vi "ni579x Write EEPROM.vi"(0 "Register Bus":refnum<class "ni579x Register Bus v1 Host.lvclass">=refnum, 1 "scope":string(combo)="characterization data eeprom", 5 "start address":u32 format="%x", 7 "data":u8[](array[numeric]) format="%x", 11 "Error In":errorcluster) -> (4 "Register Bus (out)":refnum<class "ni579x Register Bus v1 Host.lvclass">, 15 "Error Out":errorcluster)   [LabVIEW 2013]
uses:
  <instrlib>/ni579x/Register Bus/v1/Host/ni579x Register Bus v1 Host.lvclass
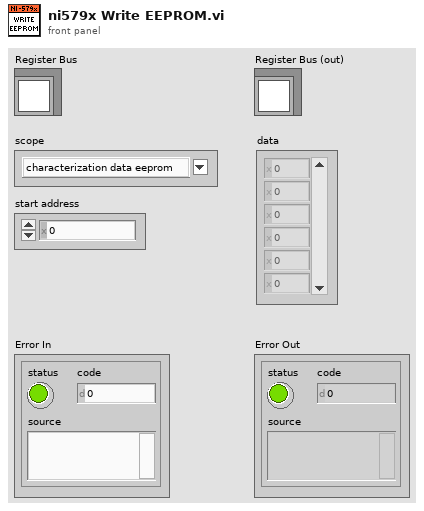
[diagram p1: front panel]
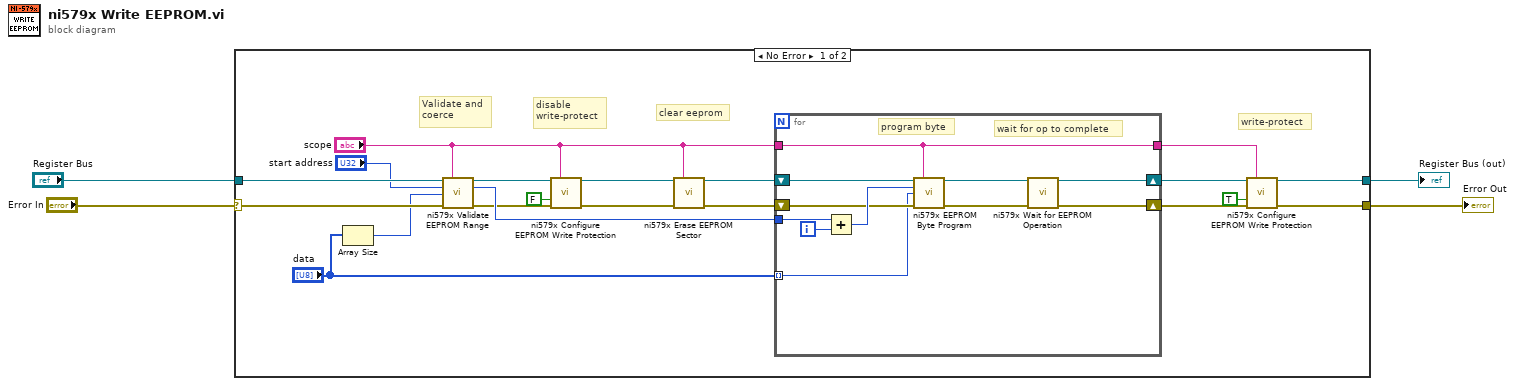
[diagram p0: block diagram]
diagram:
  n1 = case shown="No Error" "Error In" {
    selector: "Error In" -> [w22 w37]
    tunnel: [w6 w37] -> w3
    tunnel: "Register Bus" -> [w24 w36]
    tunnel: [w7 w36] -> w1
    frame No Error {
      # "write-protect"
      # "disable\nwrite-protect"
      # "clear eeprom"
      # "Validate and \ncoerce"
      n2 = Array Size(array="data") -> (size(s)=w20:i32)
      n3 = call <instrlib>:"ni579x Validate EEPROM Range.vi"("Register Bus"=w24, "scope"="scope", "start address"="start address", "size"=w20, "Error In"=w22) -> ("Register Bus (out)"=w18:refnum<class "ni579x Register Bus v1 Host.lvclass">, "coerced start address"=w21:u32, "Error Out"=w17:errorcluster)  [unwired: 7 in, 1 out]
      n4 = call <instrlib>:"ni579x Configure EEPROM Write Protection.vi"("Register Bus"=w18, "scope"="scope", "write protect?"=FALSE, "Error In"=w17) -> ("Register Bus (out)"=w15:refnum<class "ni579x Register Bus v1 Host.lvclass">, "Error Out"=w14:errorcluster)  [unwired: 10 in]
      n5 = call <instrlib>:"ni579x Erase EEPROM Sector.vi"("Register Bus"=w15, "scope"="scope", "Error In"=w14) -> ("Register Bus (out)"=w13:refnum<class "ni579x Register Bus v1 Host.lvclass">, "Error Out"=w12:errorcluster)  [unwired: 11 in]
      n6 = for {
        tunnel: w21 -> [w35]
        shift-right: [w25] -> w9
        shift-left: w12 -> [w31]
        shift-right: [w26] -> w10
        shift-left: w13 -> [w33]
        tunnel: "data" -> [w30] mode=indexing
        tunnel: "scope" -> [w29]
        tunnel: [w29] -> w5
        i -> [w34]
        # "wait for op to complete"
        # "program byte"
        n7 = Add(x=w35, y=w34) -> (x+y=w32:u32)
        n8 = call <instrlib>:"ni579x EEPROM Byte Program.vi"("Register Bus"=w33, "scope"=w29, "address"=w32, "byte"=w30, "Error In"=w31) -> ("Register Bus (out)"=w28:refnum<class "ni579x Register Bus v1 Host.lvclass">, "Error Out"=w27:errorcluster)  [unwired: 9 in]
        n9 = call <instrlib>:"ni579x Wait for EEPROM Operation.vi"("Register Bus"=w28, "Error In"=w27) -> ("Register Bus (out)"=w26:refnum<class "ni579x Register Bus v1 Host.lvclass">, "Error Out"=w25:errorcluster)  [unwired: 12 in]
      }
      n10 = call <instrlib>:"ni579x Configure EEPROM Write Protection.vi"("Register Bus"=w10, "scope"=w5, "write protect?"=TRUE, "Error In"=w9) -> ("Register Bus (out)"=w7:refnum<class "ni579x Register Bus v1 Host.lvclass">, "Error Out"=w6:errorcluster)  [unwired: 10 in]
    }
    frame Error {
    }
  }
  "Register Bus (out)" <- w1
  "Error Out" <- w3
